vi "Generate Log Record.vi"(9 "data (null)":variant, 10 "message (\"\")":string, 11 "log level":T3) -> (3 "log record":T1 {"timestamp" format="%<%x %.3X>T"})   [LabVIEW 2018, in "GLog.lvlib" / "Logger.lvclass"]
uses:
  Logger.lvclass
  Log Levels.ctl
  Log Record.ctl
  Internal Log Levels.ctl
  GLog.lvlib
panel:
  # "Connector Pane"
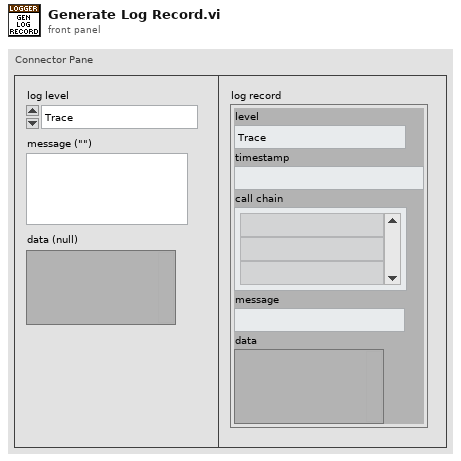
[diagram p1: front panel]
types:
  T1 = typedef "GLog.lvlib/Log Record.ctl" = cluster{"level":T2, "timestamp":timestamp, "call chain":string[], "message":string, "data":variant}
  T2 = typedef "GLog.lvlib/Internal Log Levels.ctl" = enum16{"Trace", "Debug", "Info", "Warning", "Error", "Critical", "Internal"}
  T3 = typedef "GLog.lvlib/Log Levels.ctl" = enum16{"Trace", "Debug", "Info", "Warning", "Error", "Critical"}
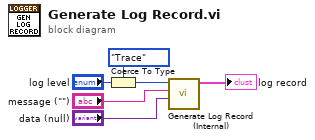
[diagram p0: block diagram]
diagram:
  n1 = Coerce To Type(0:"log level", 1:Internal_Log_Levels."Trace" ("internal log level")) -> (2:w4:T2)
  n2 = call "Generate Log Record (Internal).vi"("data (null)"="data (null)", "message (\"\")"="message (\"\")", "level (Internal)"=w4) -> ("log record"=→"log record":T1)  [unwired: 8 in]
